vi "Motor_Read_MotorSpeed.vi"(8 "error in (no error)":errorcluster, 11 "MotorControl in":refnum<class "MotorControl.lvclass">) -> (0 "error out":errorcluster, 2 "MotorEncSpeed":dbl[](array[numeric]), 3 "MotorControl out":refnum<class "MotorControl.lvclass">)   [LabVIEW 2015, in "MotorControl.lvclass"]
uses:
  MotorControl.lvclass
  MotorControl.lvclass/MotorControl.ctl
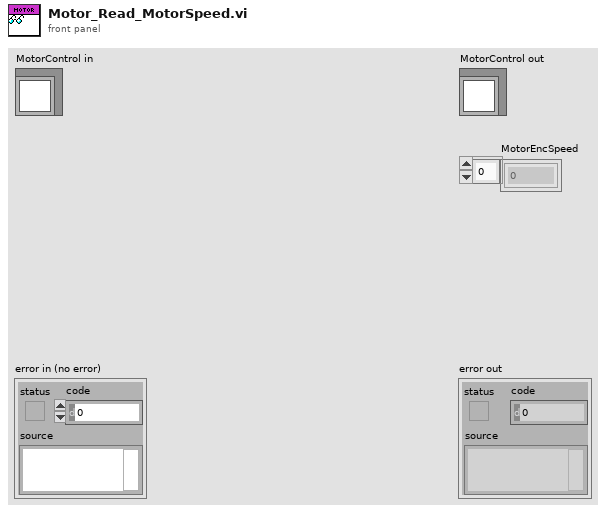
[diagram p1: front panel]
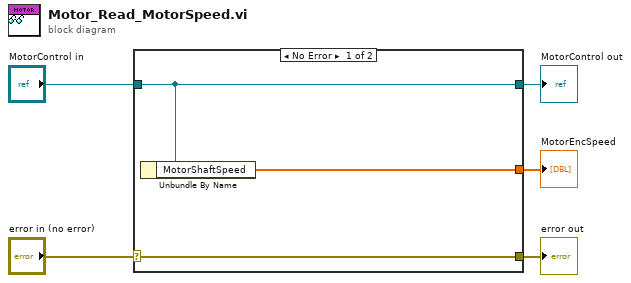
[diagram p0: block diagram]
diagram:
  n1 = case shown="No Error" "error in (no error)" {
    selector: "error in (no error)" -> [w8 w9]
    tunnel: [w8 w9] -> w4
    tunnel: [w7 w10] -> w2
    tunnel: "MotorControl in" -> [w7 w10]
    tunnel: [w6 _] -> w1
    frame No Error {
      n2 = Unbundle By Name(w7) -> ("MotorShaftSpeed"=w6:dbl[])
    }
    frame Error {
    }
  }
  "error out" <- w4
  "MotorControl out" <- w2
  "MotorEncSpeed" <- w1
